vi "Set Sender.vi"(8 "error in (no error)":errorcluster, 10 "Sender":string, 11 "Message in":refnum<class "Message.lvclass">) -> (0 "error out":errorcluster, 3 "Message out":refnum<class "Message.lvclass">)   [LabVIEW 2018, in "Application.lvlib" / "Message.lvclass"]
uses:
  Message.lvclass
  Message.lvclass/Message.ctl
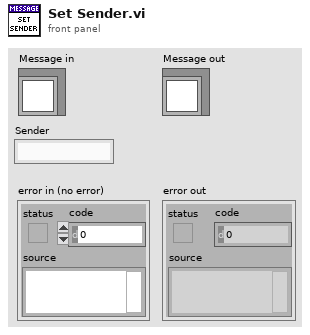
[diagram p1: front panel]
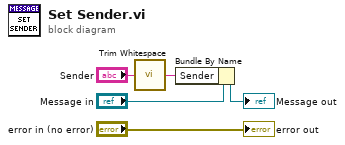
[diagram p0: block diagram]
diagram:
  n1 = call <vilib>:"Trim Whitespace.vi"("string"="Sender") -> ("trimmed string"=w1:string)  [unwired: 1 in]
  n2 = Bundle By Name(cluster="Message in", "Sender"=w1) -> (→"Message out":refnum<class "Message.lvclass">)
  "error out" <- "error in (no error)"
